vi "Save Sweep Data to csv.vi"(0 "Test Information":T2={"Exp Name"="Cold Switching", "Lot"="0233A", "Wafer"="15", "Die Type"="L22", "Die X "="6", "Die Y"="8", "Exp"="1", "Die X_Y"="8"}, 1 "Filepath":path, 3 "Selected Exp Settings":T13={"Floor_Sweep_Stop_V"=36.0, "Resistance Threshold"=1.0, "Floor_Sweep_Start_V"=36.0, "Floor_Sweep_Step_V"=1.0, "Roof_Sweep_Stop_V"=36.0, "Roof_Sweep_Start_V"=36.0, "Roof_Sweep_Step_V"=1.0, "Experiment Name"="", "Meas_Type"=[0, 2, 4]}, 5 "Date Cluster":T3, 7 "Cal Measurements":T16 {"Port 3 Capacitance" format="%#_6p"; "Port 2 Capacitance" format="%#_6p"; "Port 1 Capacitance" format="%#_6p"}, 9 "ks5080A_Meaurements":T4, 11 "Parametric Calculated Values":T5={"Voltage Calculated Values"={"P1_VPD_C"=0.0, "P2_VPD_C"=0.0, "P1_VPD_Rel_C"=0.0, "P2_VPD_Rel_C"=0.0}, "Resistance Calculated Values"={"Rc_free"=0.0, "Rc_first"=0.0, "Rc_vmax"=0.0, "Rc_last"=0.0, "Rc_end"=0.0, "VPD_R"=0.0, "VPD_Rel_R"=0.0}, "Capacitance Calculated Values"={"P1_CPD_free"=0.0, "P2_CPD_free"=0.0, "P1_CPD_vmax"=0.0, "P2_CPD_vmax"=0.0, "P1_CPD_first"=0.0, "P2_CPD_first"=0.0, "P1_CPD_last"=0.0, "P2_CPD_last"=0.0, "P1_CPD_end"=0.0, "P2_CPD_end"=0.0, "P1_CPD_max"=0.0, "P2_CPD_max "=0.0, "CPD_Free"=0.0, "CPD_First"=0.0, "CPD_max"=0.0, "CPD_Last"=0.0, "CPD_End"=0.0, "CPD_vmax"=0.0}, "Cap Calc Arrays"={"CPD_sum"=[], "P2_CPD@V"=[], "P1_CPD@V"=[], "Specific Voltages"=[32.0, 36.0]}, "Resistance Array Calc"={"RC@V"=[]}, "TN4 Calc"={"P1_TN4_ACT"=0.0, "P2_TN4_ACT "=0.0, "VPD_R_2"=0.0, "DVR"=0.0}, "Corrected_Capacitance Calculated Values"={"P1_CPD_free"=0.0, "P2_CPD_free"=0.0, "P1_CPD_vmax"=0.0, "P2_CPD_vmax"=0.0, "P1_CPD_first"=0.0, "P2_CPD_first"=0.0, "P1_CPD_last"=0.0, "P2_CPD_last"=0.0, "P1_CPD_end"=0.0, "P2_CPD_end"=0.0, "P1_CPD_max"=0.0, "P2_CPD_max "=0.0, "CPD_Free"=0.0, "CPD_First"=0.0, "CPD_max"=0.0, "CPD_Last"=0.0, "CPD_End"=0.0, "CPD_vmax"=0.0}}, 12 "Additional Data":T15, 14 "Meas Type":string="QuickView_") -> ()   [LabVIEW 2013]
uses:
  Controls/Date Control.ctl
  Controls/Test Information.ctl
  Controls/Parametric Calculated Values.ctl
  Controls/Voltage Calculated Values.ctl
  Controls/Resistance Individual Calculated Values.ctl
  Controls/Capacitance Individual Calculated Values.ctl
  Controls/Capacitance Array Calculated Values.ctl
  Controls/Resistance Array Calculated Values.ctl
  Controls/TN4 Calc.ctl
  Controls/Corrected_Capacitance Individual Calculated Values.ctl
  Controls/Additional Data.ctl
  Controls/ks5080A_Measurements.ctl
  Controls/Individual User Inputs_MultiTest.ctl
  Controls/Test Selection.ctl
  Controls/ENA_Marker Measurements.ctl
  <vilib>/Utility/file.llb/Write To Spreadsheet File (string).vi
panel:
  in  "Tab Control":T1(tab)
  # "Calculation Settings"
  # "Test Settings"
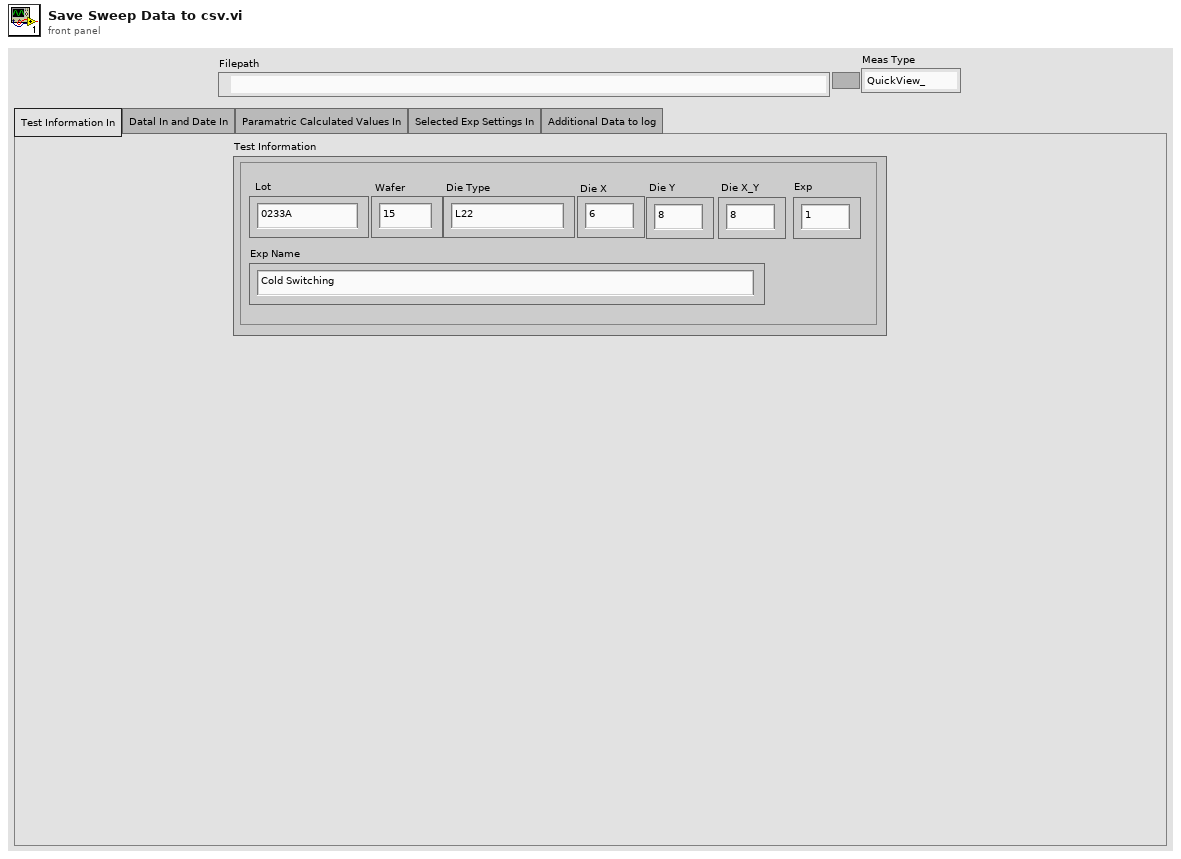
[diagram p1: front panel]
types:
  T1 = enum32{"Test Information In", "Datal In and Date In", "Paramatric Calculated Values In", "Selected Exp Settings In", "Additional Data to log"}
  T2 = typedef "Test Information.ctl" = cluster{"Exp Name":string, "Lot":string, "Wafer":string, "Die Type":string, "Die X ":string, "Die Y":string, "Exp":string, "Die X_Y":string}
  T3 = typedef "Date Control.ctl" = cluster{"Date":string, "Start Time":string, "Stop Time":string}
  T4 = typedef "ks5080A_Measurements.ctl" = cluster{"Bias_Sweep_Setting":dbl[], "Bias_voltage measurements":dbl[], "Bias_current measurements":dbl[], "P1_Capacitance":dbl[], "P2_Capacitance":dbl[], "DMM_Measurement_V":dbl[], "Contact_Source Current measurements":dbl[], "Contact_Sink Current measurements":dbl[], "Calculated_Resistance":dbl[], "P3_Capacitance":dbl[], "Port 1_S_parm":string[], "Port 2_S_parm":string[], "Port 3_S_parm":string[]}
  T5 = typedef "Parametric Calculated Values.ctl" = cluster{"Voltage Calculated Values":T6, "Resistance Calculated Values":T7, "Capacitance Calculated Values":T8, "Cap Calc Arrays":T9, "Resistance Array Calc":T10, "TN4 Calc":T11, "Corrected_Capacitance Calculated Values":T12}
  T6 = typedef "Voltage Calculated Values.ctl" = cluster{"P1_VPD_C":dbl, "P2_VPD_C":dbl, "P1_VPD_Rel_C":dbl, "P2_VPD_Rel_C":dbl}
  T7 = typedef "Resistance Individual Calculated Values.ctl" = cluster{"Rc_free":dbl, "Rc_first":dbl, "Rc_vmax":dbl, "Rc_last":dbl, "Rc_end":dbl, "VPD_R":dbl, "VPD_Rel_R":dbl}
  T8 = typedef "Capacitance Individual Calculated Values.ctl" = cluster{"P1_CPD_free":dbl, "P2_CPD_free":dbl, "P1_CPD_vmax":dbl, "P2_CPD_vmax":dbl, "P1_CPD_first":dbl, "P2_CPD_first":dbl, "P1_CPD_last":dbl, "P2_CPD_last":dbl, "P1_CPD_end":dbl, "P2_CPD_end":dbl, "P1_CPD_max":dbl, "P2_CPD_max ":dbl, "CPD_Free":dbl, "CPD_First":dbl, "CPD_max":dbl, "CPD_Last":dbl, "CPD_End":dbl, "CPD_vmax":dbl}
  T9 = typedef "Capacitance Array Calculated Values.ctl" = cluster{"CPD_sum":dbl[], "P2_CPD@V":dbl[], "P1_CPD@V":dbl[], "Specific Voltages":dbl[]}
  T10 = typedef "Resistance Array Calculated Values.ctl" = cluster{"RC@V":dbl[]}
  T11 = typedef "TN4 Calc.ctl" = cluster{"P1_TN4_ACT":dbl, "P2_TN4_ACT ":dbl, "VPD_R_2":dbl, "DVR":dbl}
  T12 = typedef "Corrected_Capacitance Individual Calculated Values.ctl" = cluster{"P1_CPD_free":dbl, "P2_CPD_free":dbl, "P1_CPD_vmax":dbl, "P2_CPD_vmax":dbl, "P1_CPD_first":dbl, "P2_CPD_first":dbl, "P1_CPD_last":dbl, "P2_CPD_last":dbl, "P1_CPD_end":dbl, "P2_CPD_end":dbl, "P1_CPD_max":dbl, "P2_CPD_max ":dbl, "CPD_Free":dbl, "CPD_First":dbl, "CPD_max":dbl, "CPD_Last":dbl, "CPD_End":dbl, "CPD_vmax":dbl}
  T13 = typedef "Individual User Inputs_MultiTest.ctl" = cluster{"Floor_Sweep_Stop_V":dbl, "Resistance Threshold":dbl, "Floor_Sweep_Start_V":dbl, "Floor_Sweep_Step_V":dbl, "Roof_Sweep_Stop_V":dbl, "Roof_Sweep_Start_V":dbl, "Roof_Sweep_Step_V":dbl, "Experiment Name":string, "Meas_Type":T14}
  T14 = typedef "Test Selection.ctl" = i32[]
  T15 = typedef "Additional Data.ctl" = cluster{"P2_Capacitance_PostTest":dbl[], "P1_Capacitance _PostTest":dbl[], "P1_Capacitance_PreTest":dbl[], "P2_Capacitance_PreTest":dbl[]}
  T16 = typedef "ENA_Marker Measurements.ctl" = cluster{"Port 1 Capacitance":dbl[], "Port 2 Capacitance":dbl[], "Port 3 Capacitance":dbl[], "Port 1_S_parm":string[], "Port 2_S_parm":string[], "Port 3_S_parm":string[]}
  T17 = enum16{"open", "replace", "create", "open or create", "replace or create", "replace or create with confirmation"}
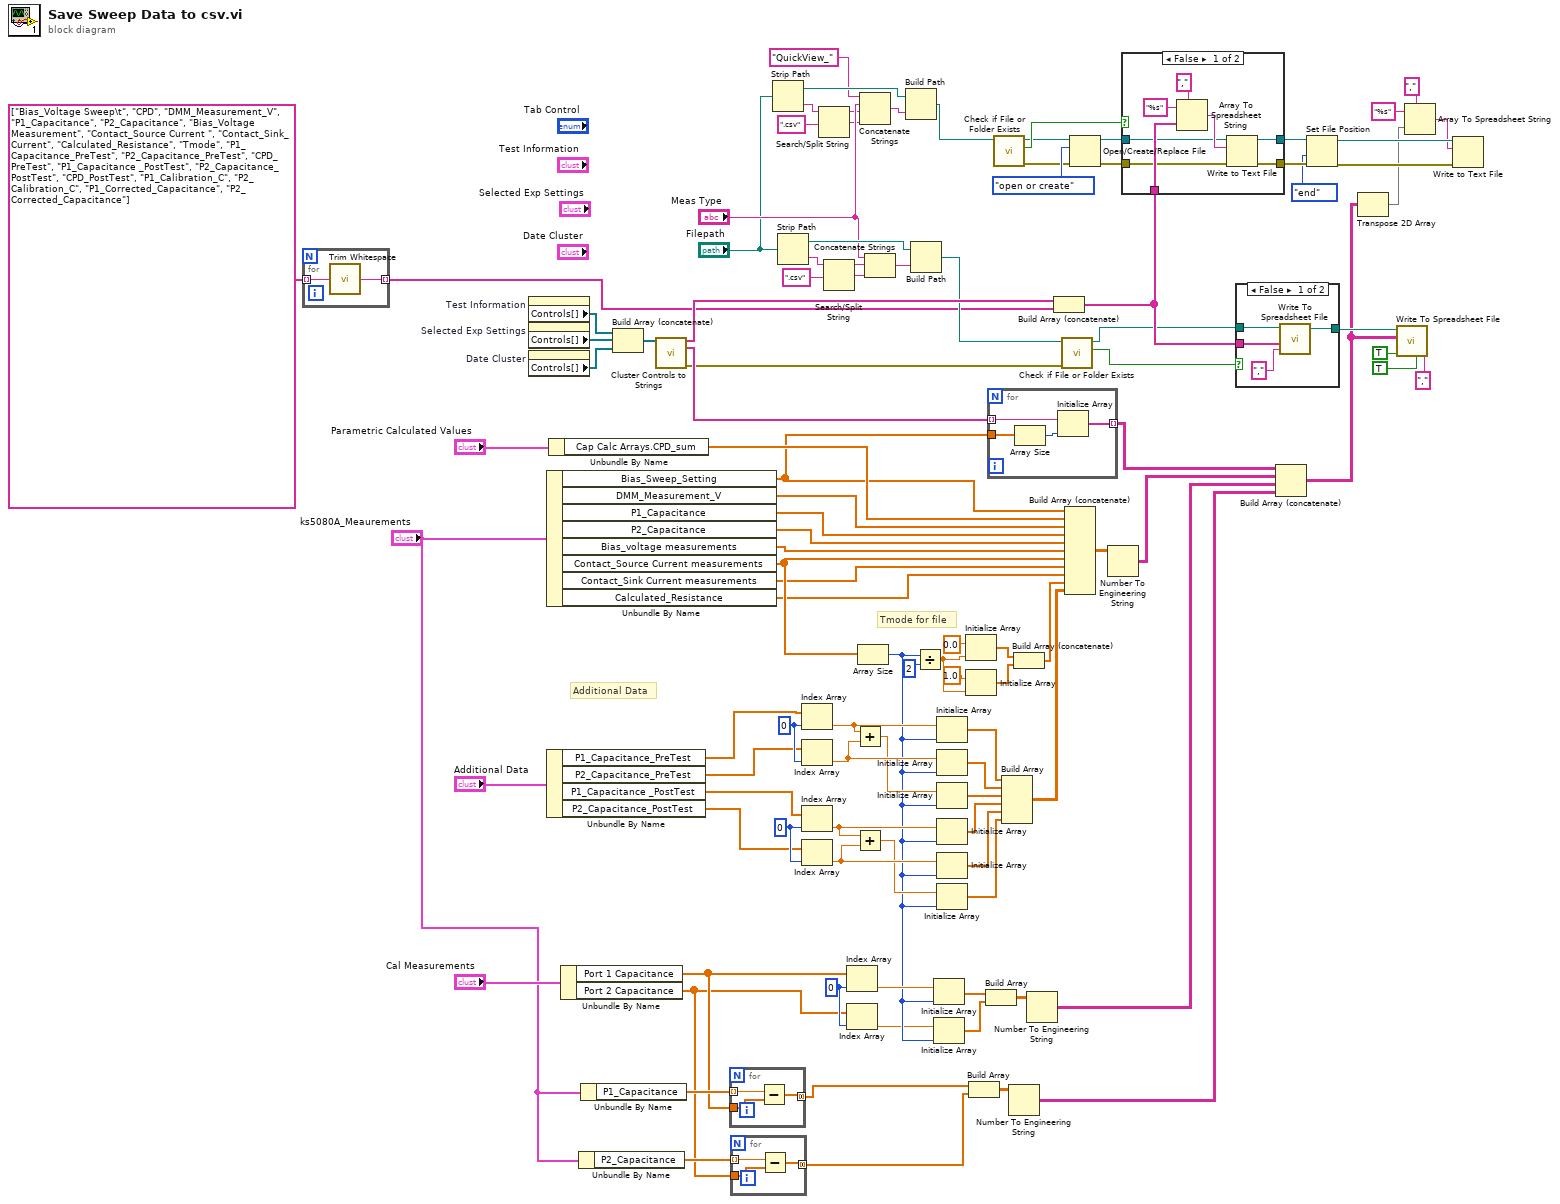
[diagram p0: block diagram]
diagram:
  w16 = 0 ("index")
  w81 = 0 ("index")
  w82 = 0 ("index")
  # "Additional Data"
  # "Tmode for file"
  n1 = for {
    tunnel: string[] ["Bias_Voltage Sweep\t", "CPD", "DMM_Measurement_V", "P1_Capacitance", "P2_Capacitance", "Bias_Voltage Measurement", "Contact_Source Current ", "Contact_Sink_Current", "Calculated_Resistance", "Tmode", "P1_Capacitance_PreTest", "P2_Capacitance_PreTest", "CPD_PreTest", "P1_Capacitance _PostTest", "P2_Capacitance_PostTest", "CPD_PostTest", "P1_Calibration_C", "P2_Calibration_C", "P1_Corrected_Capacitance", "P2_Corrected_Capacitance"] -> [w109] mode=indexing
    tunnel: [w108] -> w19 mode=indexing
    n2 = call <vilib>:"Trim Whitespace.vi"("string"=w109) -> ("trimmed string"=w108:string)  [unwired: 1 in]
  }
  n3 = property on="Test Information" class="Clust (strict)"() -> ("Controls[]"=w107:refnum<vi>[])  [unwired: 2 in, 2 out]
  n4 = property on="Selected Exp Settings" class="Clust (strict)"() -> ("Controls[]"=w21:refnum<vi>[])  [unwired: 2 in, 2 out]
  n5 = property on="Date Cluster" class="Clust (strict)"() -> ("Controls[]"=w105:refnum<vi>[])  [unwired: 2 in, 2 out]
  n6 = Unbundle By Name("ks5080A_Meaurements") -> ("Bias_Sweep_Setting"=w56:dbl[], "DMM_Measurement_V"=w55:dbl[], "P1_Capacitance"=w54:dbl[], "P2_Capacitance"=w53:dbl[], "Bias_voltage measurements"=w52:dbl[], "Contact_Source Current measurements"=w51:dbl[], "Contact_Sink Current measurements"=w50:dbl[], "Calculated_Resistance"=w49:dbl[])
  n7 = Unbundle By Name("Additional Data") -> ("P1_Capacitance_PreTest"=w66:dbl[], "P2_Capacitance_PreTest"=w65:dbl[], "P1_Capacitance _PostTest"=w64:dbl[], "P2_Capacitance_PostTest"=w63:dbl[])
  n8 = Unbundle By Name("Parametric Calculated Values") -> ("Cap Calc Arrays.CPD_sum"=w87:dbl[])
  n9 = Unbundle By Name("Cal Measurements") -> ("Port 1 Capacitance"=w7:dbl[], "Port 2 Capacitance"=w3:dbl[])
  n10 = Unbundle By Name("ks5080A_Meaurements") -> ("P2_Capacitance"=w5:dbl[])
  n11 = Unbundle By Name("ks5080A_Meaurements") -> ("P1_Capacitance"=w8:dbl[])
  n12 = Build Array (concatenate)(w107, w21, w105) -> (w106:refnum<vi>[])
  n13 = call "Cluster Controls to Strings.vi"("Controls[]"=w106) -> ("Control Labels"=w90:string[], "Control Values"=w104:string[], "Error Out"=w89:errorcluster)  [unwired: 12 in]
  n14 = for {
    tunnel: w8 -> [w112] mode=indexing
    tunnel: w7 -> [w111]
    tunnel: [w110] -> w6 mode=concatenating
    n15 = Subtract(x=w112, y=w111) -> (x-y=w110:dbl[])
  }
  n16 = for {
    tunnel: w5 -> [w115] mode=indexing
    tunnel: w3 -> [w114]
    tunnel: [w113] -> w2 mode=concatenating
    n17 = Subtract(x=w115, y=w114) -> (x-y=w113:dbl[])
  }
  n18 = Strip Path(path="Filepath") -> (stripped path=w40:path, name=w43:string)
  n19 = Strip Path(path="Filepath") -> (stripped path=w59:path, name=w62:string)
  n20 = Index Array(array=w66, index=w82) -> (element=w80:dbl)
  n21 = Index Array(array=w65, index=w82) -> (element=w79:dbl)
  n22 = Index Array(array=w64, index=w81) -> (element=w77:dbl)
  n23 = Index Array(array=w63, index=w81) -> (element=w76:dbl)
  n24 = Search/Split String(string=w43, search string/char (-)=".csv" ("search string")) -> (substring before match=w38:string, match + rest of string=w41:string)  [unwired: 1 in, 1 out]
  n25 = Search/Split String(string=w62, search string/char (-)=".csv" ("search string")) -> (substring before match=w57:string, match + rest of string=w60:string)  [unwired: 1 in, 1 out]
  n26 = Index Array(array=w7, index=w16) -> (element=w17:dbl)
  n27 = Index Array(array=w3, index=w16) -> (element=w14:dbl)
  n28 = Add(x=w80, y=w79) -> (x+y=w78:dbl)
  n29 = Add(x=w77, y=w76) -> (x+y=w75:dbl)
  n30 = Array Size(array=w51) -> (size(s)=w15:i32)
  n31 = Concatenate Strings("QuickView_" ("search string"), "Meas Type", w38, w41) -> (w39:string)
  n32 = Concatenate Strings("Meas Type", w57, w60) -> (w58:string)
  n33 = Build Path(base path=w40, name or relative path=w39) -> (appended path=w25:path)
  n34 = Build Path(base path=w59, name or relative path=w58) -> (appended path=w46:path)
  n35 = Divide(x=w15, y=2) -> (x/y=w102:dbl)
  n36 = Initialize Array(w17, w15) -> (w12:dbl[])
  n37 = Initialize Array(w14, w15) -> (w13:dbl[])
  n38 = Initialize Array(w80, w15) -> (w74:dbl[])
  n39 = Initialize Array(w79, w15) -> (w73:dbl[])
  n40 = Initialize Array(w78, w15) -> (w72:dbl[])
  n41 = Initialize Array(w77, w15) -> (w71:dbl[])
  n42 = Initialize Array(w76, w15) -> (w70:dbl[])
  n43 = Initialize Array(w75, w15) -> (w69:dbl[])
  n44 = Initialize Array(0.0, w102) -> (w103:dbl[])
  n45 = Initialize Array(1.0, w102) -> (w98:dbl[])
  n46 = Build Array(w6, w2) -> (w1:dbl[][])
  n47 = Build Array(w12, w13) -> (w11:dbl[][])
  n48 = for {
    tunnel: w56 -> [w119]
    tunnel: w104 -> [w118] mode=indexing
    tunnel: [w116] -> w93 mode=indexing
    n49 = Array Size(array=w119) -> (size(s)=w117:i32)
    n50 = Initialize Array(w118, w117) -> (w116:string[])
  }
  n51 = call <vilib>:"Check if File or Folder Exists.vi"("path"=w25) -> ("error out"=w24:errorcluster, "file or folder exists?"=w23:bool, "dup path"=w22:path)  [unwired: 8 in]
  n52 = Build Array(w74, w73, w72, w71, w70, w69) -> (w68:dbl[][])
  n53 = Number To Engineering String(4:w1) -> (0:w9:string[][])  [unwired: 3 in]
  n54 = Build Array (concatenate)(w103, w98) -> (w83:dbl[])
  n55 = Number To Engineering String(4:w11) -> (0:w10:string[][])  [unwired: 3 in]
  n56 = Build Array (concatenate)(w90, w19) -> (w85:string[])
  n57 = call <vilib>:"Check if File or Folder Exists.vi"("error in (no error)"=w89, "path"=w46) -> ("file or folder exists?"=w86:bool, "dup path"=w45:path)  [unwired: 7 in, 1 out]
  n58 = Build Array (concatenate)(w56, w87, w55, w54, w53, w52, w51, w50, w49, w83, w68) -> (w91:dbl[][])
  n59 = Open/Create/Replace File(file path (use dialog)=w22, error in=w24, operation (0:open)=T17."open or create") -> (refnum out=w37:refnum<file>, error out=w36:errorcluster)  [unwired: 3 in, 1 out]
  n60 = Number To Engineering String(4:w91) -> (0:w92:string[][])  [unwired: 3 in]
  n61 = case shown="False" w23 {
    tunnel: w85 -> [w125 _]
    tunnel: w37 -> [w123 w129]
    tunnel: w36 -> [w122 w128]
    tunnel: [w121 w128] -> w34
    tunnel: [w120 w129] -> w35
    frame False {
      n62 = Array To Spreadsheet String(delimiter (Tab)="," ("delimiter (\\t)"), array=w125, 3:"%s" ("format string")) -> (spreadsheet string=w124:string)
      n63 = Write to Text File(file (use dialog)=w123, text=w124, error in=w122) -> (refnum out=w120:refnum<file>, error out=w121:errorcluster)  [unwired: 1 in, 1 out]
    }
    frame True {
    }
  }
  n64 = case shown="False" w86 {
    tunnel: w45 -> [w133 w134]
    tunnel: w85 -> [w132 _]
    tunnel: [w130 w134] -> w97
    frame False {
      n65 = call-poly <vilib>:"Write To Spreadsheet File.vi"("delimiter (\\t)"="," ("delimiter (\\t)"), "1D data"=w132, "file path (dialog if empty)"=w133) -> ("new file path (Not A Path if cancelled)"=w130:path)  [unwired: 5 in]
    }
    frame True {
    }
  }
  n66 = Build Array (concatenate)(w93, w92, w10, w9) -> (w84:string[][])
  n67 = Set File Position(refnum=w35, from (0:start)=enum16{"start", "end", "current"}."end", error in=w34) -> (refnum out=w29:refnum<file>, error out=w30:errorcluster)  [unwired: 1 in]
  n68 = Transpose 2D Array(2D array=w84) -> (transposed array=w27:string[][])
  n69 = call-poly <vilib>:"Write To Spreadsheet File.vi"("delimiter (\\t)"="," ("delimiter (\\t)"), "transpose? (no:F)"=TRUE, "append to file? (new file:F)"=TRUE, "2D data"=w84, "file path (dialog if empty)"=w97) -> ()  [unwired: 3 in, 1 out]
  n70 = Array To Spreadsheet String(delimiter (Tab)="," ("delimiter (\\t)"), array=w27, 3:"%s" ("format string")) -> (spreadsheet string=w28:string)
  n71 = Write to Text File(file (use dialog)=w29, text=w28, error in=w30) -> ()  [unwired: 1 in, 3 out]
